vi "KnifeEdgeTestCode.vi"(6 "path":path=path "C:/Users/BOAS-USER/Documents/Data/0507/human", 7 "Init":bool, 8 "Error In":errorcluster, 9 "Z Stage":T1={"Position"=0.0, "Is.Enabled?"=TRUE, "Is.Connected?"=FALSE, "Device SN"="49876924", "AccelerationMaximum"=0.0, "VelocityMaximum"=0.0, "Acceleration"=0.0, "Velocity"=0.0, "waitTimeout (ms)"=10000, "Model"=enum."None", "Is.Homed?"=FALSE}, 10 "X Stage":T1={"Position"=0.0, "Is.Enabled?"=TRUE, "Is.Connected?"=FALSE, "Device SN"="45876539", "AccelerationMaximum"=0.0, "VelocityMaximum"=0.0, "Acceleration"=0.0, "Velocity"=0.0, "waitTimeout (ms)"=10000, "Model"=enum."None", "Is.Homed?"=FALSE}, 11 "Mosaic Paramter":T3) -> (0 "Error Out":errorcluster, 1 "Finished?":bool, 2 "Current State":T4, 3 "Current Position":cluster{"X":dbl, "Y":dbl}, 4 "size(s)":i32, 5 "Power":dbl)   [LabVIEW 2018]
uses:
  General/Controls/Go Scan Actions.ctl
  Hardware Mfg/Thorlabs Translation Stages/Controls/Translation Stage Cluster.ctl
  General/Controls/Translation Stage Types.ctl
  Hardware Mfg/Thorlabs Translation Stages/Controls/Motion Translation Module Control.ctl
  General/Controls/Set Get Controls.ctl
panel:
  in  "Average Count":i32=10 min=1 step=1
  in  "Wavelength [nm]":dbl=1300.0 caption="Wavelength (0.0)"
  in  "Avg. Time (0.0) [sec.]":dbl=0.1 caption="Average Time (0.0)" min=0.1 max=5.0 step=0.1
  out "Average Count 2":i32 caption="Average Time"
  out "Avg. Time  [sec.]":dbl caption="Average Time"
  out "Wavelength [nm] 2":dbl caption="Wavelength"
  out "Waveform Chart":dbl(graph)
  in  "No Slice?":bool
  out "XY Graph":cluster{"X":dbl, "Y":dbl}[](graph)
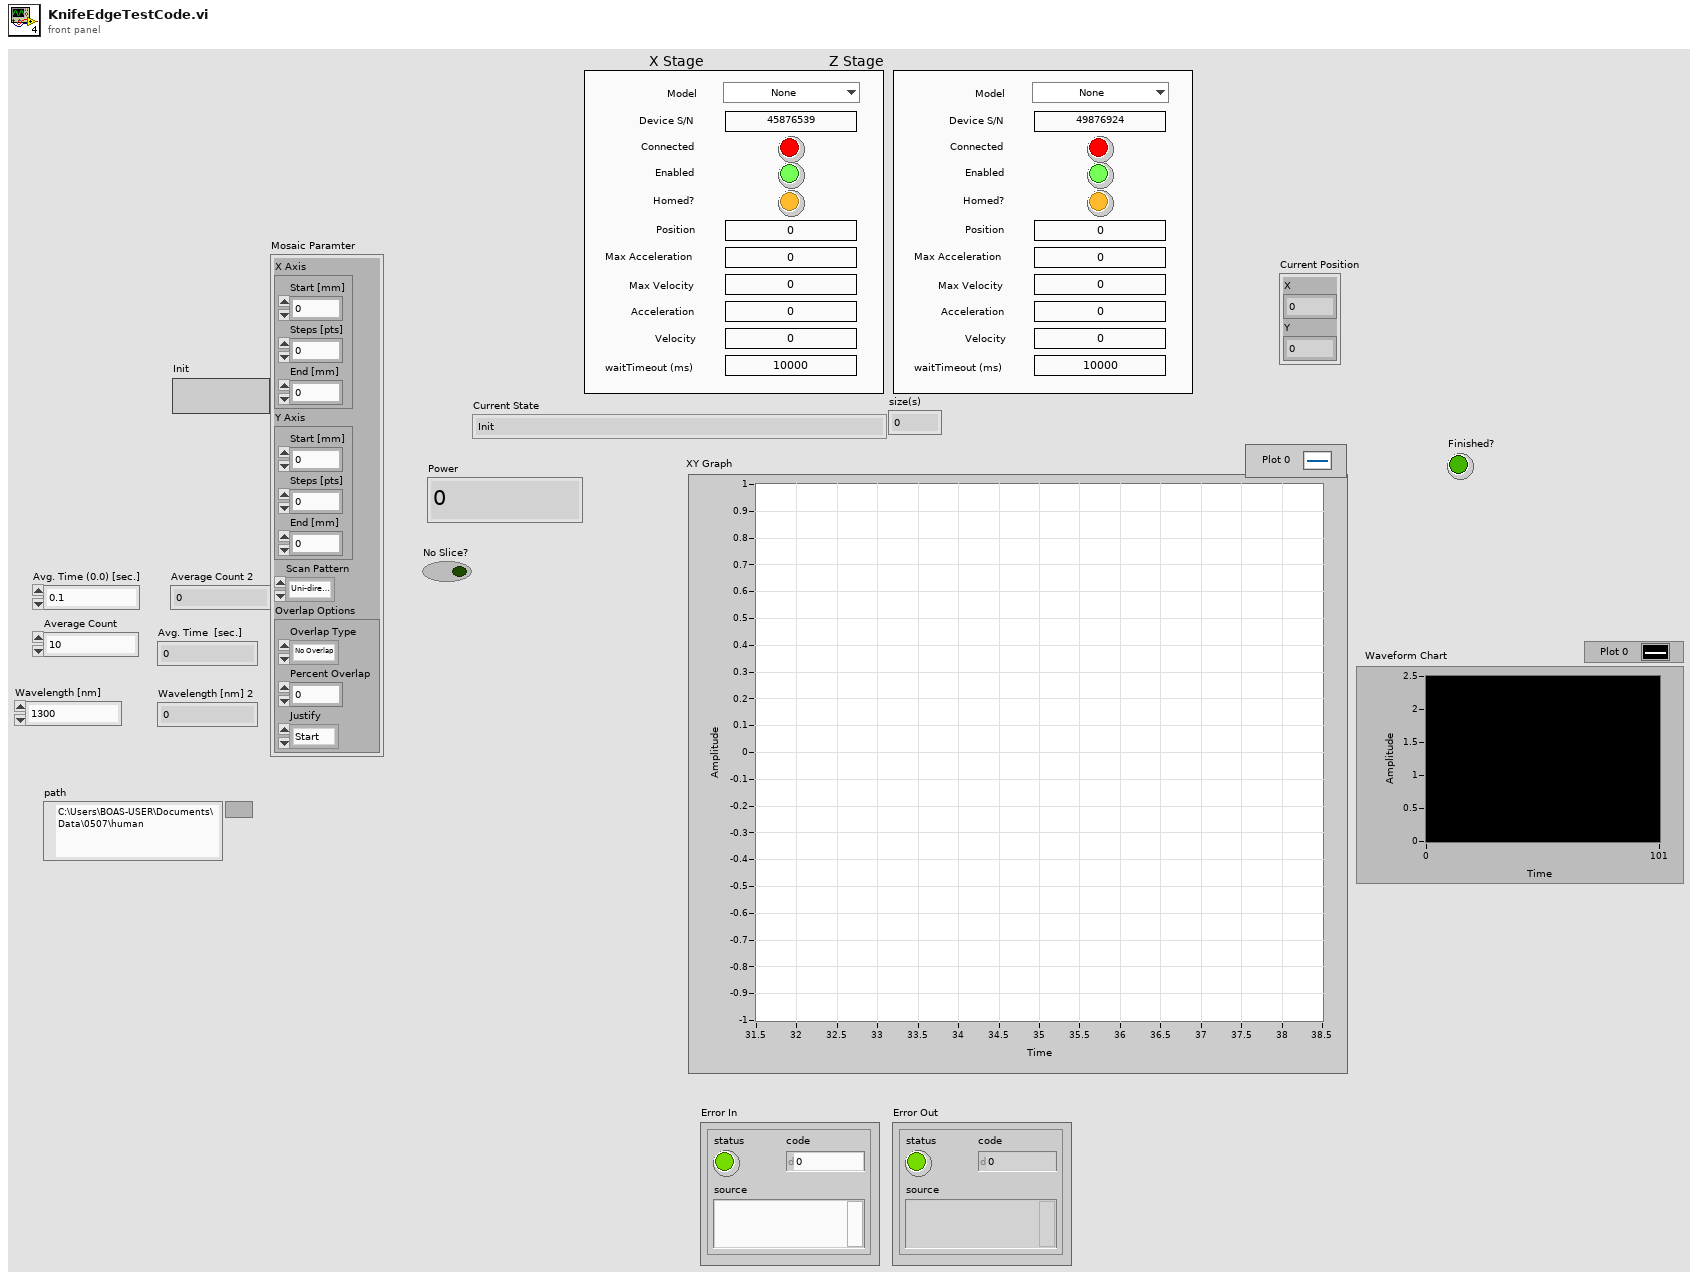
[diagram p1: front panel]
types:
  T1 = typedef "Translation Stage Cluster.ctl" = cluster{"Position":dbl, "Is.Enabled?":bool, "Is.Connected?":bool, "Device SN":string, "AccelerationMaximum":dbl, "VelocityMaximum":dbl, "Acceleration":dbl, "Velocity":dbl, "waitTimeout (ms)":i32, "Model":T2, "Is.Homed?":bool}
  T2 = typedef "Translation Stage Types.ctl" = enum16{"None", "Thorlabs LTS", "Thorlabs MLJ"}
  T3 = cluster{"X Axis":cluster{"Start [mm]":dbl, "Steps [pts]":u16, "End [mm]":dbl}, "Y Axis":cluster{"Start [mm]":dbl, "Steps [pts]":u16, "End [mm]":dbl}, "Scan Pattern":enum16{"Uni-directional", "Bi-Directional", "Spiral Out", "Spiral In"}, "Overlap Options":cluster{"Overlap Type":enum16{"No Overlap", "X Only", "Y Only", "X and Y"}, "Percent Overlap":u8, "Justify":enum16{"Start", "Center", "End"}}}
  T4 = typedef "Go Scan Actions.ctl" = enum16{"Init", "Init Scan Head", "Init Table Stage", "Init Vibratome", "Generate Mosaic", "Go Image Home", "Go Mosaic", "Acquire Image", "Go Vibratome", "Slice", "Finished"}
  T5 = typedef "Set Get Controls.ctl" = enum16{"Set", "Get"}
  T6 = typedef "Motion Translation Module Control.ctl" = enum16{"Init", "Home", "Status", "Velocity/Accel", "Position", "Jog", "Stop", "Uninit", "Enable", "Disable"}
  T7 = cluster{"Start [mm]":dbl, "Steps [pts]":u16, "End [mm]":dbl}
  T8 = cluster{"Overlap Type":enum16{"No Overlap", "X Only", "Y Only", "X and Y"}, "Percent Overlap":u8, "Justify":enum16{"Start", "Center", "End"}}
  T9 = enum16{"Uni-directional", "Bi-Directional", "Spiral Out", "Spiral In"}
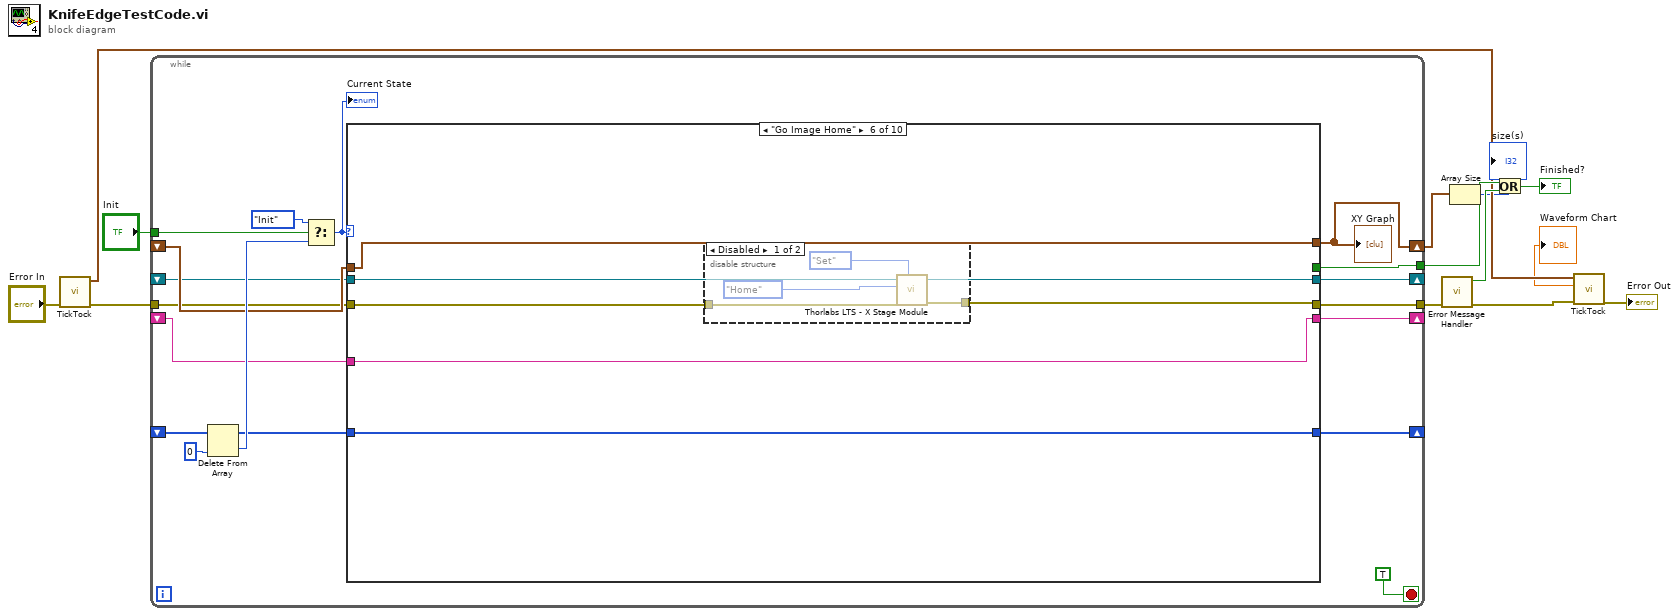
[diagram p0: block diagram]
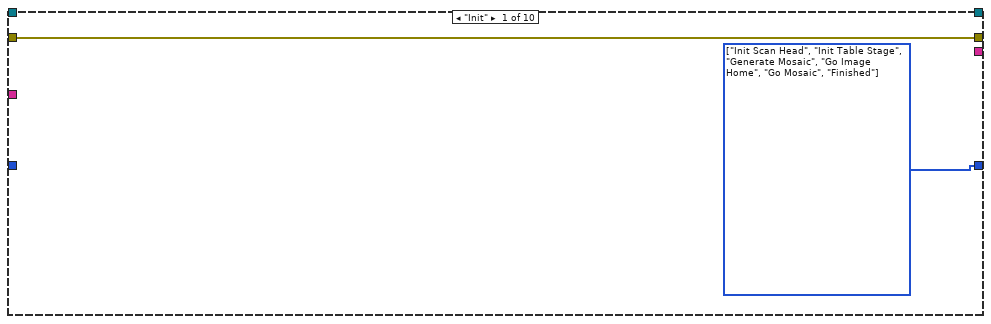
[diagram p2: hidden frame]
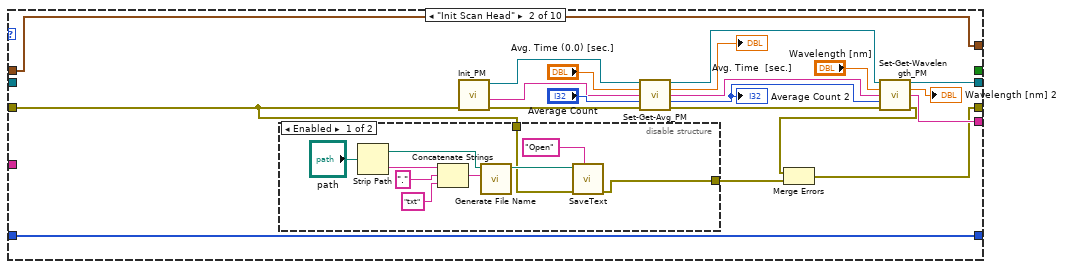
[diagram p3: hidden frame]
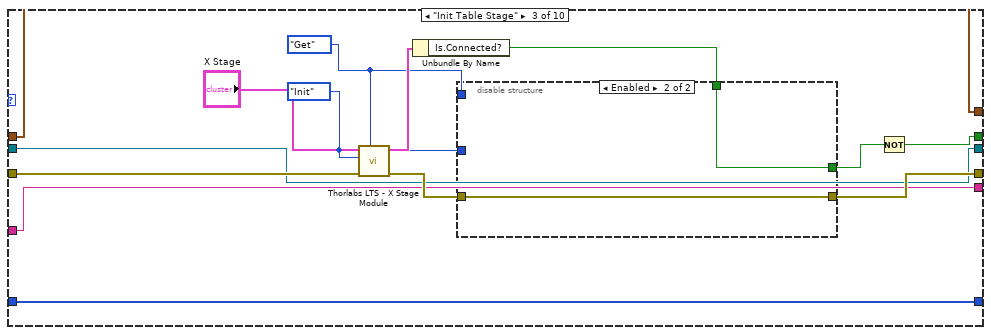
[diagram p5: hidden frame]
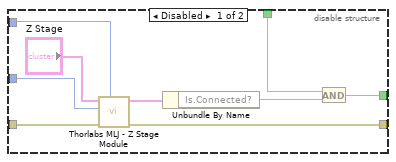
[diagram p6: hidden frame]
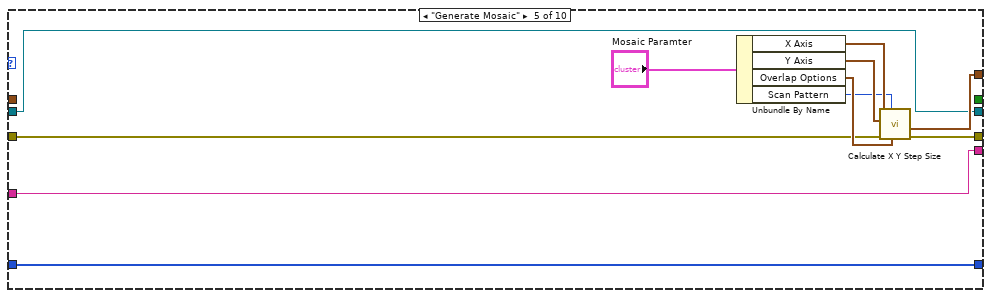
[diagram p8: hidden frame]
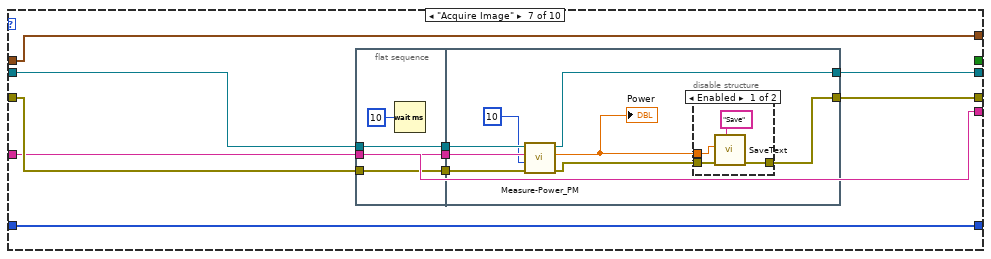
[diagram p10: hidden frame]
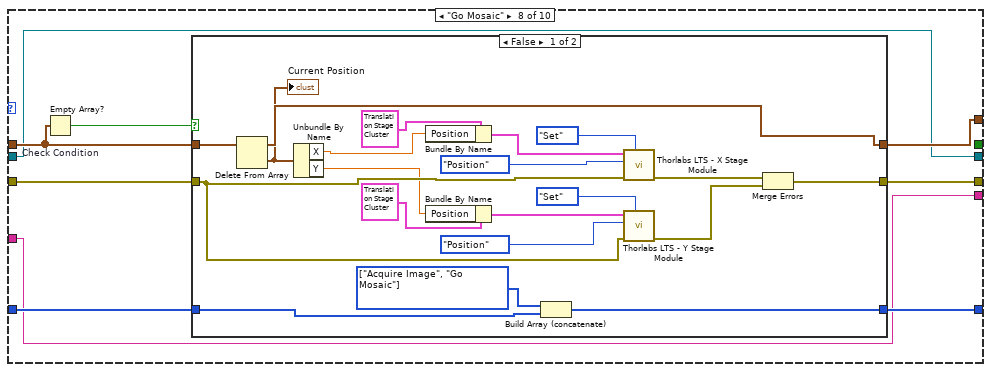
[diagram p12: hidden frame]
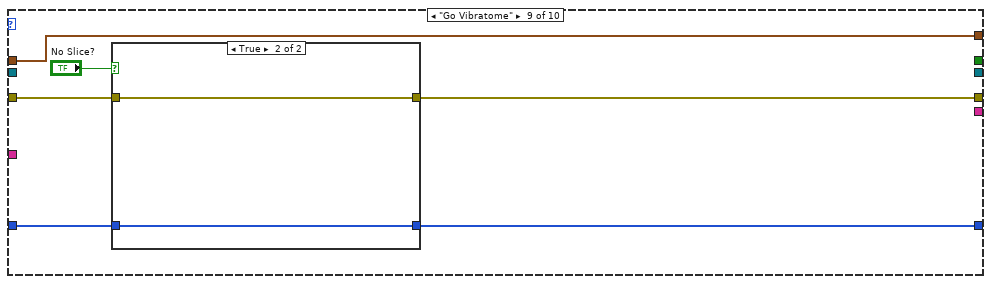
[diagram p14: hidden frame]
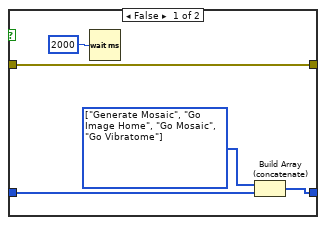
[diagram p15: hidden frame]
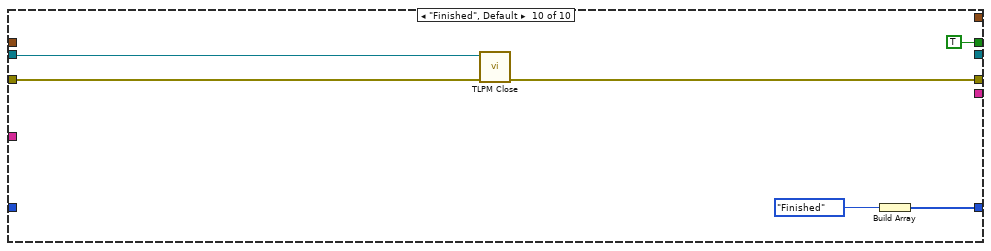
[diagram p16: hidden frame]
diagram:
  n1 = call "TickTock.vi"("Error In"="Error In") -> ("Error Out"=w7:errorcluster, "Current Time (Out)"=w5:timestamp)  [unwired: 8 in, 1 out]
  n2 = while {
    shift-right: [w27] -> _
    shift-left: _ -> [w26]
    tunnel: "Init" -> [w29]
    shift-right: [w22] -> w2
    shift-left: _ -> [w23]
    tunnel: [w21] -> w12
    tunnel: w7 -> [w19]
    tunnel: [w18] -> w11
    shift-right: [w17] -> _
    shift-left: _ -> [w15]
    shift-right: [w16] -> _
    shift-left: _ -> [w14]
    stop <- TRUE stop-if-true
    n3 = Delete From Array(array=w26, index=0) -> (deleted portion=w25:T4, array with subset deleted=w24:T4[])  [unwired: 1 in]
    n4 = Select(t=Go_Scan_Actions."Init", s=w29, f=w25) -> (s? t:f=w28:T4)
    "Current State" <- w28
    n5 = case shown="\"Go Image Home\"" w28 {
      tunnel: [w32 w52 w76 w92 w104 w109 w123 w146 w176 w191] -> w27
      tunnel: w24 -> [_ w52 w76 w92 w104 w109 w123 w147 w177 _]
      tunnel: [_ w53 w77 w93 w103 w110 w124 w150 w179 _] -> w22
      tunnel: w23 -> [_ w53 w77 w93 _ w110 w124 w149 w179 _]
      tunnel: [_ _ w71 _ _ _ _ _ _ TRUE] -> w21
      tunnel: w19 -> [w33 w37 w75 w91 w97 w106 w121 w145 w175 w189]
      tunnel: [w33 w35 w69 w91 w96 w105 w118 w144 w174 w188] -> w18
      tunnel: [_ w39 w65 w89 w94 w107 w119 w143 _ _] -> w17
      tunnel: [_ w38 w64 w90 w95 w108 w120 w142 _ _] -> w16
      tunnel: w15 -> [_ _ w65 w89 w94 w107 w119 w143 _ _]
      tunnel: w14 -> [_ _ w64 w90 w95 w108 w122 w142 _ w187]
      frame "Init" {
        w32 = T4[] [enum."Init Scan Head", enum."Init Table Stage", enum."Generate Mosaic", enum."Go Image Home", enum."Go Mosaic", enum."Finished"] items=["Init", "Init Scan Head", "Init Table Stage", "Init Vibratome", "Generate Mosaic", "Go Image Home", "Go Mosaic", "Acquire Image", "Go Vibratome", "Slice", "Finished"]
      }
      frame "Init Scan Head" {
        n6 = disable-structure shown="Enabled" {
          disable-tunnel: w37 -> [w55 _]
          disable-tunnel: [w54 _] -> w36
          frame Enabled {
            n7 = Strip Path(path="path") -> (stripped path=w60:path, name=w61:string)
            n8 = Concatenate Strings(w61, "." ("string"), "txt" ("string")) -> (w59:string)
            n9 = call "Generate File Name.vi"("name or relative path"=w59, "base path"=w60) -> ("appended path"=w57:path)  [unwired: 9 in]
            n10 = call "SaveText.vi"("action"="Open", "error in"=w55, "file path (use dialog)"=w57) -> ("error out"=w54:errorcluster)  [unwired: 8 in]
          }
          frame Disabled {
          }
        }
        n11 = call "Init_PM.vi"("error in (no error)"=w37) -> ("error out"=w40:errorcluster, "Sensor Name"=w41:string, "instrument handle out"=w42:refnum<visa-resource-name>)  [unwired: 8 in]
        n12 = call "Set-Get-Avg_PM.vi"("instrument handle"=w42, "Average Time (0.0)"="Avg. Time (0.0) [sec.]", "Sensor"=w41, "Average Count"="Average Count", "error in (no error)"=w40) -> ("instrument handle out"=w49:refnum<visa-resource-name>, "Average Time"=→"Avg. Time  [sec.]":dbl, "Sensor 2"=w47:string, "Average Count"=w46:i32, "error out"=w50:errorcluster)  [unwired: 6 in]
        "Average Count 2" <- w46
        n13 = call "Set-Get-Wavelength_PM.vi"("instrument handle"=w49, "Wavelength"="Wavelength [nm]", "Sensor Name"=w47, "Average Count"=w46, "error in (no error)"=w50) -> ("instrument handle out"=w38:refnum<visa-resource-name>, "Wavelength"=→"Wavelength [nm] 2":dbl, "Sensor Name 2"=w39:string, "error out"=w34:errorcluster)  [unwired: 6 in, 1 out]
        n14 = Merge Errors(w34, w36) -> (w35:errorcluster)
      }
      frame "Init Table Stage" {
        w66 = Set_Get_Controls."Get" ("Set/Get")
        w68 = Motion_Translation_Module_Control."Init" ("Action")
        n15 = call "Thorlabs LTS - X Stage Module.vi"("Set/Get"=w66, "Error In"=w75, "Action"=w68, "Cluster In"="X Stage") -> ("Error Out"=w74:errorcluster, "Cluster Out"=w73:T1)  [unwired: 6 in]
        n16 = Unbundle By Name(w73) -> ("Is.Connected?"=w72:bool)
        n17 = disable-structure shown="Enabled" {
          disable-tunnel: w74 -> [w86 w87]
          disable-tunnel: w72 -> [w85 w88]
          disable-tunnel: [w84 w87] -> w69
          disable-tunnel: w68 -> [w82 _]
          disable-tunnel: [w80 w88] -> w67
          disable-tunnel: w66 -> [w78 _]
          frame Disabled {
            n18 = call "Thorlabs MLJ - Z Stage Module.vi"("Set/Get"=w78, "Error In"=w86, "Action"=w82, "Cluster In"="Z Stage") -> ("Error Out"=w84:errorcluster, "Cluster Out"=w81:T1)  [unwired: 6 in]
            n19 = Unbundle By Name(w81) -> ("Is.Connected?"=w79:bool)
            n20 = And(x=w85, y=w79) -> (x .and. y?=w80:bool)
          }
          frame Enabled {
          }
        }
        n21 = Not(x=w67) -> (.not. x?=w71:bool)
      }
      frame "Init Vibratome" {
      }
      frame "Generate Mosaic" {
        n22 = Unbundle By Name("Mosaic Paramter") -> ("X Axis"=w101:T7, "Y Axis"=w100:T7, "Overlap Options"=w99:T8, "Scan Pattern"=w98:T9)
        n23 = call "Calculate X Y Step Size.vi"("Overlap Options"=w99, "Scan Pattern"=w98, "Error In"=w97, "Y Axis"=w100, "X Axis"=w101) -> ("Error Out"=w96:errorcluster, "Array"=w103:cluster{"X":dbl, "Y":dbl}[])  [unwired: 3 in, 2 out]
      }
      frame "Go Image Home" {
        n24 = disable-structure shown="Disabled" {
          disable-tunnel: w106 -> [w112 _]
          disable-tunnel: [w111 _] -> w105
          frame Disabled {
            n25 = call "Thorlabs LTS - X Stage Module.vi"("Set/Get"=Set_Get_Controls."Set", "Error In"=w112, "Action"=Motion_Translation_Module_Control."Home") -> ("Error Out"=w111:errorcluster)  [unwired: 7 in, 1 out]
          }
          frame Enabled {
          }
        }
      }
      frame "Acquire Image" {
        n26 = flat-sequence {
          tunnel: w119 -> [w126]
          tunnel: w121 -> [w127]
          tunnel: w122 -> [w128]
          tunnel: [w128] -> w117
          tunnel: [w127] -> w116
          tunnel: [w126] -> w115
          tunnel: [w134] -> w120
          tunnel: [w132] -> w118
          tunnel: w117 -> [w136]
          tunnel: w116 -> [w135]
          tunnel: w115 -> [w133]
          frame #0 {
            n27 = Wait (ms)(milliseconds to wait=u32 10) -> ()  [unwired: 1 out]
          }
          frame #1 {
            n28 = call "Measure-Power_PM.vi"("error in (no error)"=w135, "Numeric"=10, "Sensor"=w133, "instrument handle"=w136) -> ("error out"=w130:errorcluster, "Power"=w129:dbl, "instrument handle out"=w134:refnum<visa-resource-name>)  [unwired: 5 in]
            "Power" <- w129
            n29 = disable-structure shown="Enabled" {
              disable-tunnel: [w140 w141] -> w132
              disable-tunnel: w130 -> [w139 w141]
              disable-tunnel: w129 -> [w137 _]
              frame Enabled {
                n30 = call "SaveText.vi"("action"="Save", "error in"=w139, "data in"=w137) -> ("error out"=w140:errorcluster)  [unwired: 8 in]
              }
              frame Disabled {
              }
            }
          }
        }
      }
      frame "Go Mosaic" {
        n31 = Empty Array? "Check Condition"(array=w149) -> (empty?=w148:bool)
        n32 = case shown="False" w148 {
          tunnel: [w170 w173] -> w150
          tunnel: w149 -> [w169 w173]
          tunnel: w147 -> [w168 w172]
          tunnel: [w166 w172] -> w146
          tunnel: w145 -> [w156 w171]
          tunnel: [w152 w171] -> w144
          frame False {
            w165 = T4[] [enum."Acquire Image", enum."Go Mosaic"] items=["Init", "Init Scan Head", "Init Table Stage", "Init Vibratome", "Generate Mosaic", "Go Image Home", "Go Mosaic", "Acquire Image", "Go Vibratome", "Slice", "Finished"]
            n33 = Delete From Array(array=w169) -> (deleted portion=w167:cluster{"X":dbl, "Y":dbl}, array with subset deleted=w170:cluster{"X":dbl, "Y":dbl}[])  [unwired: 2 in]
            "Current Position" <- w167
            n34 = Unbundle By Name(w167) -> ("X"=w160:dbl, "Y"=w154:dbl)
            n35 = Bundle By Name(cluster=T1 {"Position"=0.0, "Is.Enabled?"=FALSE, "Is.Connected?"=FALSE, "Device SN"="45876539", "AccelerationMaximum"=0.0, "VelocityMaximum"=0.0, "Acceleration"=0.0, "Velocity"=0.0, "waitTimeout (ms)"=10000, "Model"=enum."None", "Is.Homed?"=FALSE} ("Cluster In"), "Position"=w160) -> (w159:T1)
            n36 = Bundle By Name(cluster=T1 {"Position"=0.0, "Is.Enabled?"=FALSE, "Is.Connected?"=FALSE, "Device SN"="45876539", "AccelerationMaximum"=0.0, "VelocityMaximum"=0.0, "Acceleration"=0.0, "Velocity"=0.0, "waitTimeout (ms)"=10000, "Model"=enum."None", "Is.Homed?"=FALSE} ("Cluster In"), "Position"=w154) -> (w153:T1)
            n37 = Build Array (concatenate)(w165, w168) -> (w166:T4[])
            n38 = call "Thorlabs LTS - X Stage Module.vi"("Set/Get"=Set_Get_Controls."Set", "Error In"=w156, "Action"=Motion_Translation_Module_Control."Position", "Cluster In"=w159) -> ("Error Out"=w163:errorcluster)  [unwired: 6 in, 1 out]
            n39 = call "Thorlabs LTS - Y Stage Module.vi"("Set/Get"=Set_Get_Controls."Set", "Error In"=w156, "Action"=Motion_Translation_Module_Control."Position", "Cluster In"=w153) -> ("Error Out"=w151:errorcluster)  [unwired: 6 in, 1 out]
            n40 = Merge Errors(w163, w151) -> (w152:errorcluster)
          }
          frame True {
          }
        }
      }
      frame "Go Vibratome" {
        n41 = case shown="True" "No Slice?" {
          tunnel: w177 -> [w184 w186]
          tunnel: [w183 w186] -> w176
          tunnel: w175 -> [w180 w185]
          tunnel: [w180 w185] -> w174
          frame False {
            w182 = T4[] [enum."Generate Mosaic", enum."Go Image Home", enum."Go Mosaic", enum."Go Vibratome"] items=["Init", "Init Scan Head", "Init Table Stage", "Init Vibratome", "Generate Mosaic", "Go Image Home", "Go Mosaic", "Acquire Image", "Go Vibratome", "Slice", "Finished"]
            n42 = Wait (ms)(milliseconds to wait=u32 2000) -> ()  [unwired: 1 out]
            n43 = Build Array (concatenate)(w182, w184) -> (w183:T4[])
          }
          frame True {
          }
        }
      }
      frame "Finished", Default {
        n44 = call "TLPM Close.vi"("error in (no error)"=w189, "instrument handle"=w187) -> ("error out"=w188:errorcluster)  [unwired: 9 in]
        n45 = Build Array(Go_Scan_Actions."Finished") -> (w191:T4[])
      }
    }
    "XY Graph" <- w22
  }
  n46 = call "Error Message Handler.vi"("Error In"=w11) -> ("Error Out"=w3:errorcluster, "T button?"=w9:bool)  [unwired: 9 in]
  n47 = Array Size(array=w2) -> (size(s)=→"size(s)":i32)
  n48 = Or(x=w12, y=w9) -> (x .or. y?=→"Finished?":bool)
  n49 = call "TickTock.vi"("Error In"=w3, "Current Time (In)"=w5) -> ("Error Out"=→"Error Out":errorcluster, "dt"=→"Waveform Chart":dbl)  [unwired: 7 in, 1 out]
